vi "Esclavo.vi"() -> ()   [LabVIEW 2017]
uses:
  <vilib>/Modbus/slave/Create Slave Instance (TCP).vi
  <vilib>/Modbus/slave/Modbus Slave.lvclass
panel:
  in  "stop":bool
  out "coil values":bool[](array[boolean])
  out "register values":u16[](array[numeric])
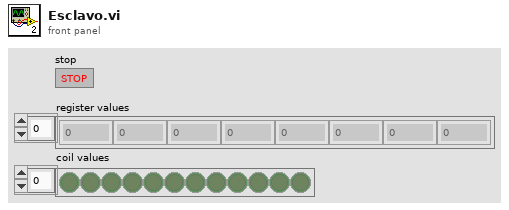
[diagram p1: front panel]
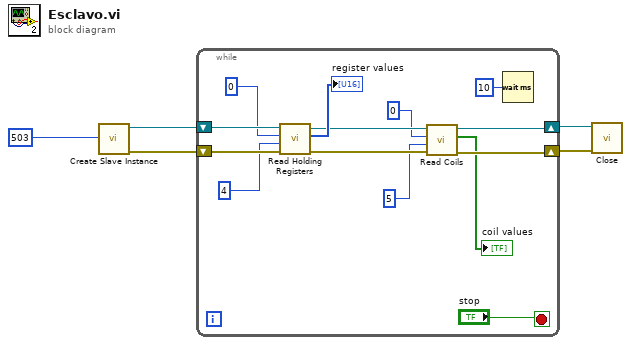
[diagram p0: block diagram]
diagram:
  n1 = call-poly <vilib>:"Create Slave Instance.vi"("port (502)"=u16 503) -> ("error out"=w4:errorcluster, "TCP slave instance"=w3:refnum<class "Modbus Slave.lvclass">)  [unwired: 9 in]
  n2 = while {
    shift-right: [w10] -> w1
    shift-left: w3 -> [w18]
    shift-right: [w9] -> w2
    shift-left: w4 -> [w19]
    stop <- "stop" stop-if-true
    n3 = call-dynamic "Read Holding Registers.vi"("error in (no error)"=w19, "number of holding registers"=u16 4, "starting address"=u16 0, "Modbus slave in"=w18) -> ("error out"=w13:errorcluster, "register values"=→"register values":u16[], "Modbus slave out"=w14:refnum<class "Modbus Slave.lvclass">)  [unwired: 5 in]
    n4 = call-dynamic "Read Coils.vi"("error in (no error)"=w13, "number of coils"=u16 5, "starting address"=u16 0, "Modbus slave in"=w14) -> ("error out"=w9:errorcluster, "coil values"=→"coil values":bool[], "Modbus slave out"=w10:refnum<class "Modbus Slave.lvclass">)  [unwired: 5 in]
    n5 = Wait (ms)(milliseconds to wait=u32 10) -> ()  [unwired: 1 out]
  }
  n6 = call-dynamic "Close.vi"("error in (no error)"=w2, "Modbus slave in"=w1) -> ()  [unwired: 9 in, 1 out]
